vi "Sudo GUID.vi"() -> (5 "GUID String":string)   [LabVIEW 2018]
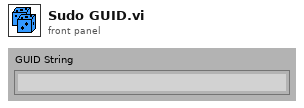
[diagram p1: front panel]
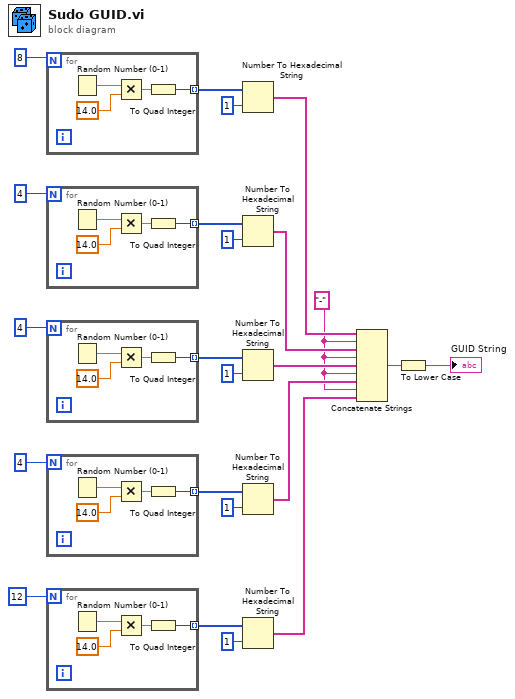
[diagram p0: block diagram]
diagram:
  w2 = "-"
  n1 = for {
    N: 8 -> [_]
    tunnel: [w24] -> w22 mode=indexing
    n2 = Random Number (0-1)() -> (number: 0 to 1=w27:dbl)
    n3 = Multiply(x=w27, y=14.0) -> (x*y=w25:dbl)
    n4 = To Quad Integer(1:w25) -> (0:w24:i64)
  }
  n5 = for {
    N: 4 -> [_]
    tunnel: [w28] -> w19 mode=indexing
    n6 = Random Number (0-1)() -> (number: 0 to 1=w31:dbl)
    n7 = Multiply(x=w31, y=14.0) -> (x*y=w29:dbl)
    n8 = To Quad Integer(1:w29) -> (0:w28:i64)
  }
  n9 = for {
    N: 4 -> [_]
    tunnel: [w32] -> w16 mode=indexing
    n10 = Random Number (0-1)() -> (number: 0 to 1=w35:dbl)
    n11 = Multiply(x=w35, y=14.0) -> (x*y=w33:dbl)
    n12 = To Quad Integer(1:w33) -> (0:w32:i64)
  }
  n13 = for {
    N: 4 -> [_]
    tunnel: [w36] -> w13 mode=indexing
    n14 = Random Number (0-1)() -> (number: 0 to 1=w39:dbl)
    n15 = Multiply(x=w39, y=14.0) -> (x*y=w37:dbl)
    n16 = To Quad Integer(1:w37) -> (0:w36:i64)
  }
  n17 = for {
    N: 12 -> [_]
    tunnel: [w40] -> w10 mode=indexing
    n18 = Random Number (0-1)() -> (number: 0 to 1=w43:dbl)
    n19 = Multiply(x=w43, y=14.0) -> (x*y=w41:dbl)
    n20 = To Quad Integer(1:w41) -> (0:w40:i64)
  }
  n21 = Number To Hexadecimal String(1:i16 1 ("width (-)"), 2:w22) -> (0:w8:string[])
  n22 = Number To Hexadecimal String(1:i16 1 ("width (-)"), 2:w19) -> (0:w7:string[])
  n23 = Number To Hexadecimal String(1:i16 1 ("width (-)"), 2:w16) -> (0:w6:string[])
  n24 = Number To Hexadecimal String(1:i16 1 ("width (-)"), 2:w13) -> (0:w5:string[])
  n25 = Number To Hexadecimal String(1:i16 1 ("width (-)"), 2:w10) -> (0:w4:string[])
  n26 = Concatenate Strings(w8, w2, w7, w2, w6, w2, w5, w2, w4) -> (w3:string)
  n27 = To Lower Case(string=w3) -> (all lower case string=→"GUID String":string)
